vi "Alarm UI.vi"(9 "Alarm Reason in":string, 10 "Alarm in":bool=TRUE, 11 "Alarm DVR":refnum<data-value>) -> ()   [LabVIEW 2018, in "Alarm.lvclass"]
uses:
  Alarm.lvclass
  Alarm.lvclass/Alarm.ctl
  Set Alarm Reason.vi
panel:
  out "Alarm Reason":string
  out "Alarm":bool=TRUE
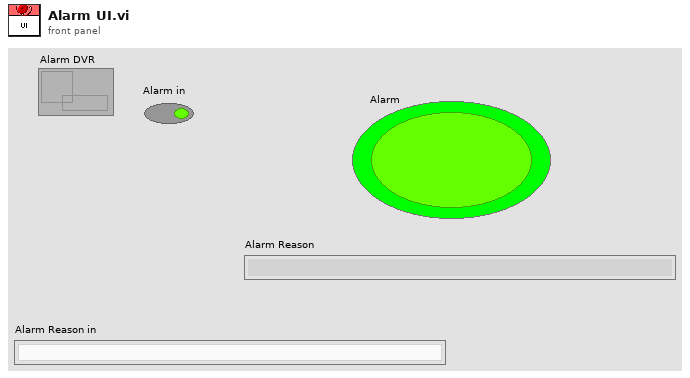
[diagram p1: front panel]
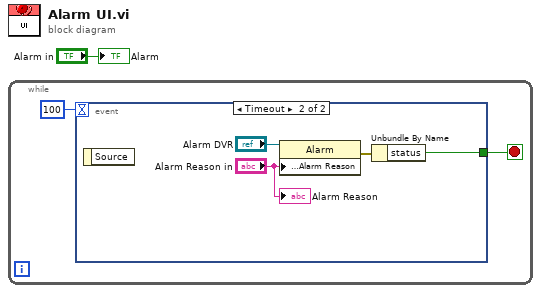
[diagram p0: block diagram]
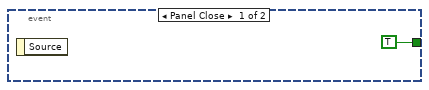
[diagram p2: hidden frame]
diagram:
  n1 = while {
    stop <- w3 stop-if-true
    n2 = event shown="[1] Timeout" {
      selector: _ -> [_ _]
      dyn-events: _ -> [_ _]
      timeout: 100 -> [_ _]
      tunnel: [TRUE w5] -> w3
      event Panel Close {
        n3 = event-data() -> ()  [unwired: 1 in, 1 out]
      }
      event Timeout {
        n4 = event-data() -> ()  [unwired: 1 in, 1 out]
        n5 = property class="Alarm"(reference="Alarm DVR", "Accessors:Alarm Reason"="Alarm Reason in") -> (error out=w7:errorcluster)  [unwired: 1 in, 1 out]
        n6 = Unbundle By Name(w7) -> ("status"=w5:bool)
        "Alarm Reason" <- "Alarm Reason in"
      }
    }
  }
  "Alarm" <- "Alarm in"
